vi "toXml.vi"(8 "error in (no error)":errorcluster, 11 "ScriptEventList in":refnum<class "ScriptEventList.lvclass">) -> (0 "error out":errorcluster, 2 "event_listXml":refnum<class "xmlNode.lvclass">, 3 "ScriptEventList out":refnum<class "ScriptEventList.lvclass">)   [LabVIEW 2009, in "Tools.lvlib" / "Scripting.lvlib" / "ScriptEventList.lvclass"]
uses:
  ScriptEventList.lvclass
  xmlNode/xmlNode.lvclass
  ScriptEventList.lvclass/ScriptEventList.ctl
  ScriptEvent.lvclass
  ScriptEvents/Ramp/RampEvent/RampEvent.lvclass
  ScriptEvents/SingleTone/SingleTone.lvclass
  ScriptEvents/Rf Event/rf.lvclass
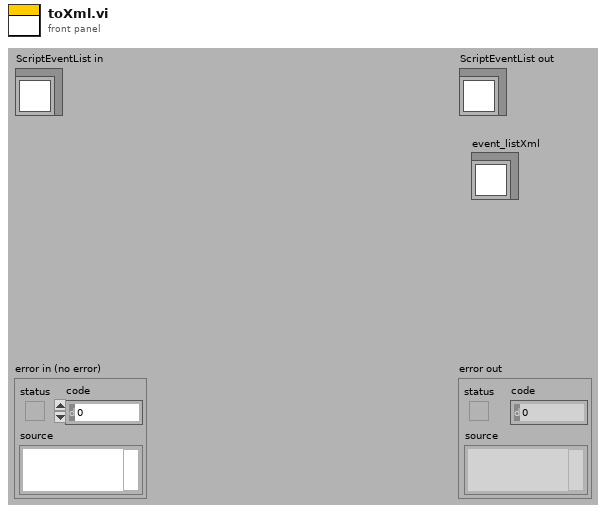
[diagram p1: front panel]
types:
  T1 = enum16{"changeValue", "pulse", "clock", "rampUp", "rampDown", "singleTone", "singleToneRamp", "playFile", "rf", "rfRamp", "delay"}
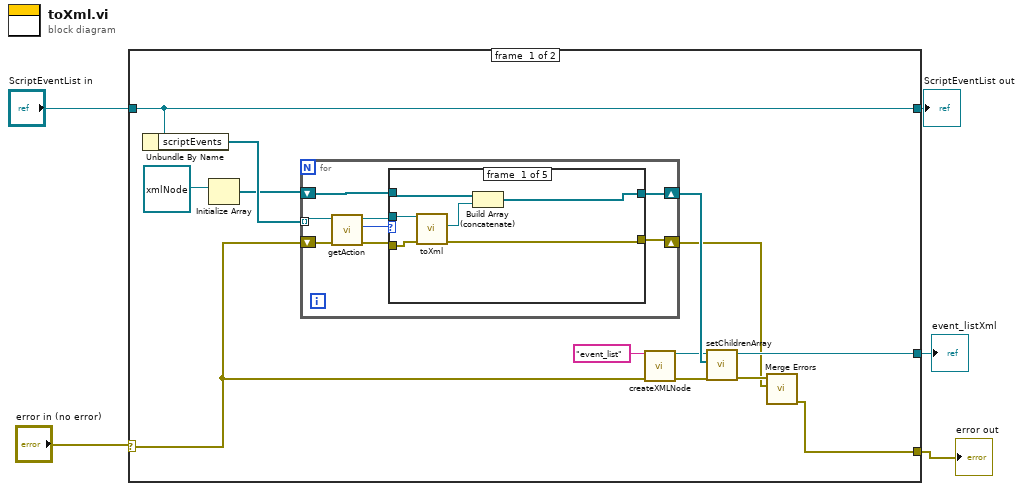
[diagram p0: block diagram]
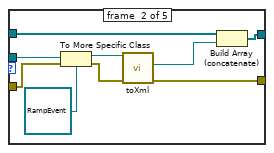
[diagram p2: hidden frame]
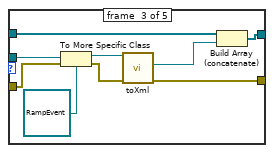
[diagram p3: hidden frame]
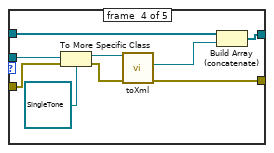
[diagram p4: hidden frame]
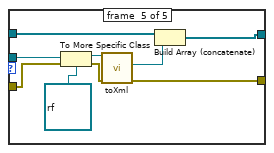
[diagram p5: hidden frame]
diagram:
  n1 = case shown="No Error" "error in (no error)" {
    selector: "error in (no error)" -> [w11 w70]
    tunnel: [w7 w70] -> w4
    tunnel: [w18 w69] -> w2
    tunnel: "ScriptEventList in" -> [w18 w69]
    tunnel: [w14 _] -> w1
    frame #0 {
      n2 = Unbundle By Name(w18) -> ("scriptEvents"=w17:refnum<class "ScriptEvent.lvclass">[])
      n3 = Initialize Array(refnum<class "xmlNode.lvclass"> refnum ("Tools.lvlib:xml.lvlib:xmlNode.lvclass")) -> (w16:refnum<class "xmlNode.lvclass">[])  [unwired: 1 in]
      n4 = for {
        tunnel: w17 -> [w26] mode=indexing
        shift-right: [w19] -> w15
        shift-left: w16 -> [w21]
        shift-right: [w22] -> w8
        shift-left: w11 -> [w23]
        n5 = call "getAction.vi"("error in (no error)"=w23, "ScriptEvent.lvclass in"=w26) -> ("error out"=w20:errorcluster, "action"=w25:T1, "ScriptEvent.lvclass out"=w24:refnum<class "ScriptEvent.lvclass">)  [unwired: 7 in]
        n6 = case shown="\"changeValue\", Default" w25 {
          tunnel: w21 -> [w32 w34 w43 w53 w62]
          tunnel: w24 -> [w31 w40 w49 w59 w68]
          tunnel: w20 -> [w30 w39 w48 w58 w67]
          tunnel: [w29 w35 w44 w54 w63] -> w22
          tunnel: [w27 w33 w42 w52 w61] -> w19
          frame #0 {
            n7 = call-dynamic "toXml.vi"("error in (no error)"=w30, "ScriptEvent in"=w31) -> ("error out"=w29:errorcluster, "scriptEventXML"=w28:refnum<class "xmlNode.lvclass">)  [unwired: 7 in, 1 out]
            n8 = Build Array (concatenate)(w32, w28) -> (w27:refnum<class "xmlNode.lvclass">[])
          }
          frame #1 {
            n9 = To More Specific Class(target class=refnum<class "RampEvent.lvclass"> refnum ("Tools.lvlib:Scripting.lvlib:RampEvent.lvclass"), reference=w40, error in=w39) -> (specific class reference=w38:refnum<class "RampEvent.lvclass">, error out=w37:errorcluster)
            n10 = call-dynamic "toXml.vi"("error in (no error)"=w37, "RampEvent in"=w38) -> ("error out"=w35:errorcluster, "scriptEventXML"=w36:refnum<class "xmlNode.lvclass">)  [unwired: 7 in, 1 out]
            n11 = Build Array (concatenate)(w34, w36) -> (w33:refnum<class "xmlNode.lvclass">[])
          }
          frame #2 {
            n12 = To More Specific Class(target class=refnum<class "RampEvent.lvclass"> refnum ("Tools.lvlib:Scripting.lvlib:RampEvent.lvclass"), reference=w49, error in=w48) -> (specific class reference=w47:refnum<class "RampEvent.lvclass">, error out=w46:errorcluster)
            n13 = call-dynamic "toXml.vi"("error in (no error)"=w46, "RampEvent in"=w47) -> ("error out"=w44:errorcluster, "scriptEventXML"=w45:refnum<class "xmlNode.lvclass">)  [unwired: 7 in, 1 out]
            n14 = Build Array (concatenate)(w43, w45) -> (w42:refnum<class "xmlNode.lvclass">[])
          }
          frame #3 {
            n15 = To More Specific Class(target class=refnum<class "SingleTone.lvclass"> refnum ("Tools.lvlib:Scripting.lvlib:SingleTone.lvclass"), reference=w59, error in=w58) -> (specific class reference=w57:refnum<class "SingleTone.lvclass">, error out=w56:errorcluster)
            n16 = call-dynamic "toXml.vi"("error in (no error)"=w56, "SingleTone in"=w57) -> ("error out"=w54:errorcluster, "scriptEventXML"=w55:refnum<class "xmlNode.lvclass">)  [unwired: 7 in, 1 out]
            n17 = Build Array (concatenate)(w53, w55) -> (w52:refnum<class "xmlNode.lvclass">[])
          }
          frame #4 {
            n18 = To More Specific Class(target class=refnum<class "rf.lvclass"> refnum ("Tools.lvlib:Scripting.lvlib:rf.lvclass"), reference=w68, error in=w67) -> (specific class reference=w66:refnum<class "rf.lvclass">, error out=w65:errorcluster)
            n19 = call-dynamic "toXml.vi"("error in (no error)"=w65, "rf in"=w66) -> ("error out"=w63:errorcluster, "scriptEventXML"=w64:refnum<class "xmlNode.lvclass">)  [unwired: 7 in, 1 out]
            n20 = Build Array (concatenate)(w62, w64) -> (w61:refnum<class "xmlNode.lvclass">[])
          }
        }
      }
      n21 = call "createXMLNode.vi"("error in (no error)"=w11, "name"="event_list") -> ("error out"=w12:errorcluster, "xmlNode out"=w13:refnum<class "xmlNode.lvclass">)  [unwired: 8 in]
      n22 = call-dynamic "setChildrenArray.vi"("error in (no error)"=w12, "Children"=w15, "xmlNode.lvclass in"=w13) -> ("error out"=w9:errorcluster, "xmlNode.lvclass out"=w14:refnum<class "xmlNode.lvclass">)  [unwired: 7 in]
      n23 = call <vilib>:"Merge Errors.vi"("error in 2 (no error)"=w8, "error in 1 (no error)"=w9) -> ("error out"=w7:errorcluster)  [unwired: 5 in]
    }
    frame #1 {
    }
  }
  "error out" <- w4
  "ScriptEventList out" <- w2
  "event_listXml" <- w1
